vi "Radio Rx Tx Test.vi"(4 "Powers":string[](array[string]), 6 "Channels":string[](array[string]), 7 "Test to Run":enum16{"TX", "RX"}(ring), 8 "error in (no error)":errorcluster, 9 "Packets":i32, 10 "Test Radio in":refnum<class "SC Manufacturing Test.lvclass">, 11 "SC Manufacturing Test in":refnum<class "SC Manufacturing Test.lvclass">) -> (0 "error out":errorcluster, 3 "Passed":bool)   [LabVIEW 2015, in "MTS Radio Test.lvclass"]
uses:
  MTS Radio Test.lvclass
  Classes/Manufacturing Test/Class/SC Manufacturing Test.lvclass
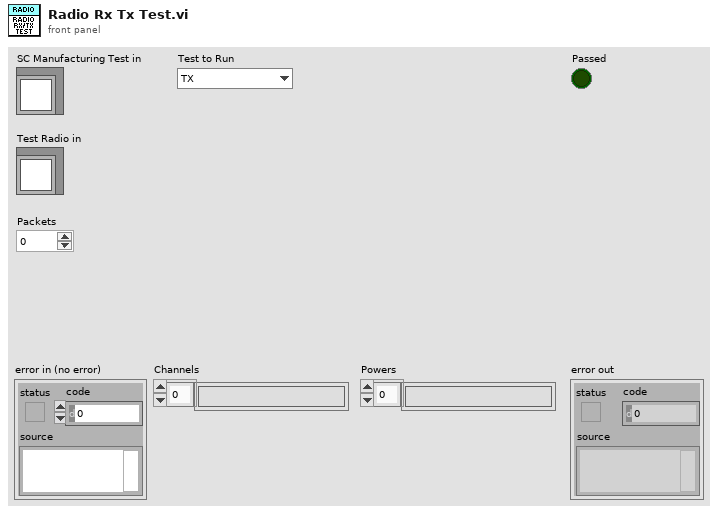
[diagram p1: front panel]
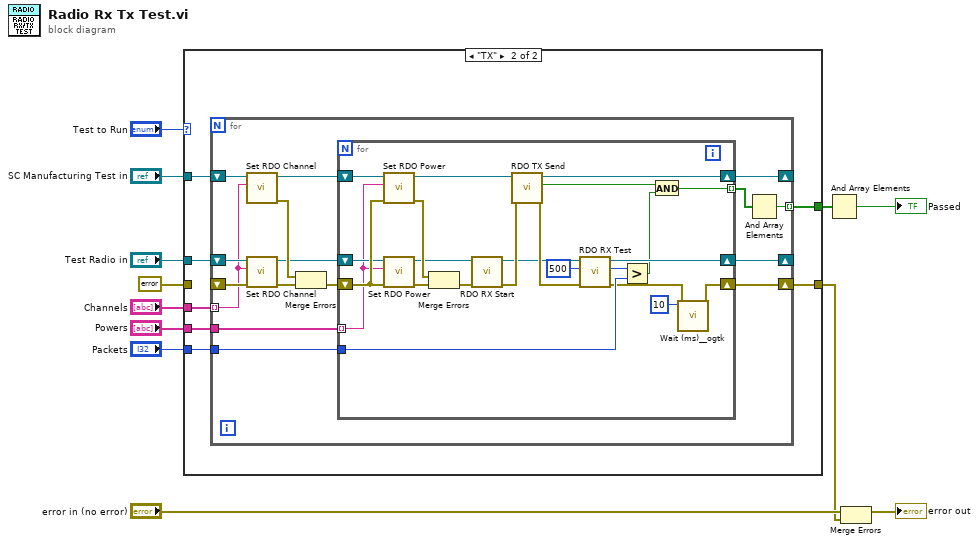
[diagram p0: block diagram]
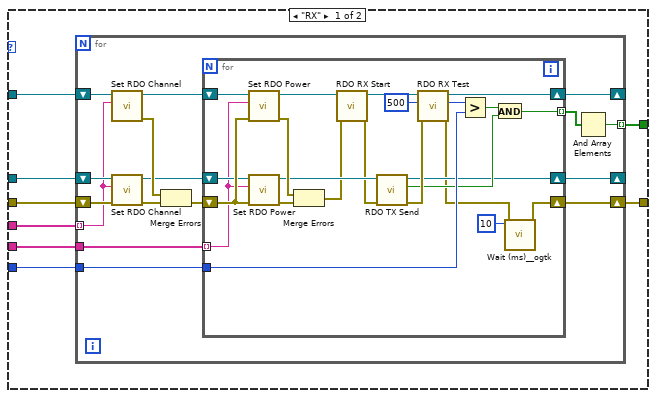
[diagram p2: hidden frame]
diagram:
  n1 = case shown="\"TX\"" "Test to Run" {
    tunnel: [w14 w66] -> w1
    tunnel: "Channels" -> [w18 w65]
    tunnel: "Packets" -> [w16 w64]
    tunnel: "Powers" -> [w17 w63]
    tunnel: [w15 w62] -> w8
    tunnel: "SC Manufacturing Test in" -> [w20 w61]
    tunnel: "Test Radio in" -> [w19 w60]
    tunnel: errorcluster {"status"=FALSE, "code"=0, "source"=""} ("error IO") -> [w13 _]
    frame "RX" {
      n2 = for {
        shift-right: [w34] -> _
        shift-left: w20 -> [w33]
        shift-right: [w27] -> _
        shift-left: w19 -> [w31]
        tunnel: w18 -> [w29] mode=indexing
        tunnel: w17 -> [w28]
        tunnel: w16 -> [w21]
        tunnel: [w25] -> w15 mode=indexing
        shift-right: [w24] -> w14
        shift-left: w13 -> [w35]
        n3 = call "Set RDO Channel.vi"("Channel"=w29, "Acrobat Template in"=w33) -> ("error out"=w36:errorcluster, "Acrobat Template out"=w32:refnum<class "SC Manufacturing Test.lvclass">)  [unwired: 8 in]
        n4 = call "Set RDO Channel.vi"("error in (no error)"=w35, "Channel"=w29, "Acrobat Template in"=w31) -> ("error out"=w23:errorcluster, "Acrobat Template out"=w30:refnum<class "SC Manufacturing Test.lvclass">)  [unwired: 7 in]
        n5 = Merge Errors(w36, w23) -> (w22:errorcluster)
        n6 = for {
          shift-right: [w40] -> w34
          shift-left: w32 -> [w55]
          shift-right: [w42] -> w27
          shift-left: w30 -> [w56]
          tunnel: w28 -> [w54] mode=indexing
          tunnel: w21 -> [w52]
          tunnel: [w51] -> w26 mode=indexing
          shift-right: [w37] -> w24
          shift-left: w22 -> [w58]
          n7 = call "Set RDO Power.vi"("error in (no error)"=w58, "Power"=w54, "Acrobat Template in"=w55) -> ("error out"=w59:errorcluster, "Acrobat Template out"=w49:refnum<class "SC Manufacturing Test.lvclass">)  [unwired: 7 in]
          n8 = call "Set RDO Power.vi"("error in (no error)"=w58, "Power"=w54, "Acrobat Template in"=w56) -> ("error out"=w50:errorcluster, "Acrobat Template out"=w48:refnum<class "SC Manufacturing Test.lvclass">)  [unwired: 7 in]
          n9 = Merge Errors(w59, w50) -> (w46:errorcluster)
          n10 = call "RDO RX Start.vi"("error in (no error)"=w46, "Acrobat Template in"=w49) -> ("error out"=w47:errorcluster, "Acrobat Template out"=w41:refnum<class "SC Manufacturing Test.lvclass">)  [unwired: 8 in]
          n11 = call "RDO TX Send.vi"("error in (no error)"=w47, "Acrobat Template in"=w48) -> ("error out"=w45:errorcluster, "Passed"=w43:bool, "Acrobat Template out"=w42:refnum<class "SC Manufacturing Test.lvclass">)  [unwired: 7 in]
          n12 = call "RDO RX Test.vi"("error in (no error)"=w45, "Time to Wait (2000 ms)"=u32 500, "Acrobat Template in"=w41) -> ("error out"=w38:errorcluster, "Packets Received"=w53:i32, "Acrobat Template out"=w40:refnum<class "SC Manufacturing Test.lvclass">)  [unwired: 5 in, 1 out]
          n13 = Greater?(x=w53, y=w52) -> (0:w44:bool)
          n14 = And(x=w44, y=w43) -> (x .and. y?=w51:bool)
          n15 = call <userlib>:"Wait (ms)__ogtk.vi"("error in (no error)"=w38, "milliseconds to wait"=u32 10) -> ("error out"=w37:errorcluster)  [unwired: 8 in, 1 out]
        }
        n16 = And Array Elements(Boolean array=w26) -> (logical AND=w25:bool)
      }
    }
    frame "TX" {
      n17 = for {
        shift-right: [w80] -> _
        shift-left: w61 -> [w79]
        shift-right: [w72] -> _
        shift-left: w60 -> [w77]
        tunnel: w65 -> [w75] mode=indexing
        tunnel: w63 -> [w74]
        tunnel: w64 -> [w73]
        tunnel: [w70] -> w62 mode=indexing
        shift-right: [w69] -> w66
        shift-left: _ -> [w82]
        n18 = call "Set RDO Channel.vi"("Channel"=w75, "Acrobat Template in"=w79) -> ("error out"=w81:errorcluster, "Acrobat Template out"=w78:refnum<class "SC Manufacturing Test.lvclass">)  [unwired: 8 in]
        n19 = call "Set RDO Channel.vi"("error in (no error)"=w82, "Channel"=w75, "Acrobat Template in"=w77) -> ("error out"=w68:errorcluster, "Acrobat Template out"=w76:refnum<class "SC Manufacturing Test.lvclass">)  [unwired: 7 in]
        n20 = Merge Errors(w81, w68) -> (w67:errorcluster)
        n21 = for {
          shift-right: [w101] -> w80
          shift-left: w78 -> [w96]
          shift-right: [w92] -> w72
          shift-left: w76 -> [w98]
          tunnel: w74 -> [w94] mode=indexing
          tunnel: w73 -> [w89]
          tunnel: [w88] -> w71 mode=indexing
          shift-right: [w83] -> w69
          shift-left: w67 -> [w102]
          n22 = call "Set RDO Power.vi"("error in (no error)"=w102, "Power"=w94, "Acrobat Template in"=w96) -> ("error out"=w105:errorcluster, "Acrobat Template out"=w95:refnum<class "SC Manufacturing Test.lvclass">)  [unwired: 7 in]
          n23 = call "Set RDO Power.vi"("error in (no error)"=w102, "Power"=w94, "Acrobat Template in"=w98) -> ("error out"=w86:errorcluster, "Acrobat Template out"=w97:refnum<class "SC Manufacturing Test.lvclass">)  [unwired: 7 in]
          n24 = Merge Errors(w105, w86) -> (w87:errorcluster)
          n25 = call "RDO RX Start.vi"("error in (no error)"=w87, "Acrobat Template in"=w97) -> ("error out"=w103:errorcluster, "Acrobat Template out"=w100:refnum<class "SC Manufacturing Test.lvclass">)  [unwired: 8 in]
          n26 = call "RDO TX Send.vi"("error in (no error)"=w103, "Acrobat Template in"=w95) -> ("error out"=w104:errorcluster, "Passed"=w91:bool, "Acrobat Template out"=w101:refnum<class "SC Manufacturing Test.lvclass">)  [unwired: 7 in]
          n27 = call "RDO RX Test.vi"("error in (no error)"=w104, "Time to Wait (2000 ms)"=u32 500, "Acrobat Template in"=w100) -> ("error out"=w84:errorcluster, "Packets Received"=w93:i32, "Acrobat Template out"=w92:refnum<class "SC Manufacturing Test.lvclass">)  [unwired: 5 in, 1 out]
          n28 = Greater?(x=w93, y=w89) -> (0:w90:bool)
          n29 = And(x=w91, y=w90) -> (x .and. y?=w88:bool)
          n30 = call <userlib>:"Wait (ms)__ogtk.vi"("error in (no error)"=w84, "milliseconds to wait"=u32 10) -> ("error out"=w83:errorcluster)  [unwired: 8 in, 1 out]
        }
        n31 = And Array Elements(Boolean array=w71) -> (logical AND=w70:bool)
      }
    }
  }
  n32 = And Array Elements(Boolean array=w8) -> (logical AND=→"Passed":bool)
  n33 = Merge Errors("error in (no error)", w1) -> (→"error out":errorcluster)
